vi "zad2.vi"() -> ()   [LabVIEW 2025]
panel:
  out "Numeric":dbl
  out "x+y":dbl
  out "Array":dbl[](array[numeric])
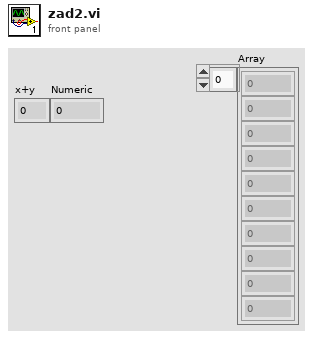
[diagram p1: front panel]
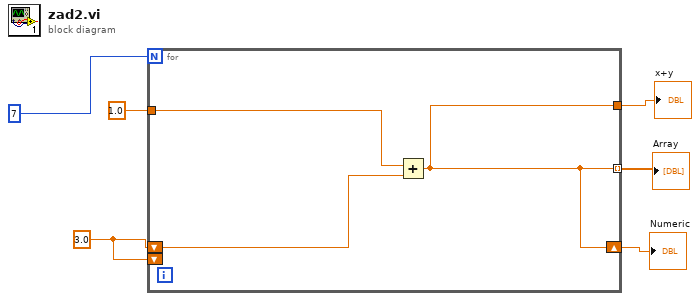
[diagram p0: block diagram]
diagram:
  w5 = 3.0
  n1 = for {
    N: 7 ("dimension size") -> [_]
    shift-right: [w7] -> w1
    shift-left: w5 -> [w9]
    tunnel: [w7] -> w6 mode=indexing
    shift-left: w5 -> [_]
    tunnel: 1.0 ("element") -> [w8]
    tunnel: [w7] -> w2
    n2 = Add(x=w8, y=w9) -> (x+y=w7:dbl)
  }
  "Array" <- w6
  "x+y" <- w2
  "Numeric" <- w1
